vi "Read Msg Input.vi"(11 "Stopped Msg in":refnum<class "Stopped Msg.lvclass">) -> (2 "Msg Input":refnum<class "Msg Input.lvclass">)   [LabVIEW 2020, in "jettl.lvlib" / "Stopped jettl Msg.lvlib" / "Stopped Msg.lvlib" / "Stopped Msg.lvclass"]
uses:
  Stopped Msg.lvclass
  Msg Input/Msg Input.lvclass
  Stopped Msg.lvclass/Stopped Msg.ctl
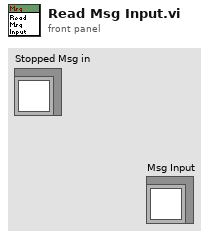
[diagram p1: front panel]
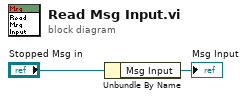
[diagram p0: block diagram]
diagram:
  n1 = Unbundle By Name("Stopped Msg in") -> ("Msg Input"=→"Msg Input":refnum<class "Msg Input.lvclass">)
